vi "Wait for stop mMc Edited.vi"(5 "Controller #":string, 6 "wait for in pos":bool, 7 "Port":T1={"P type"=0, "reference"="", " Terminator "="\r\n", "Timeout"=300} {"Timeout" step=10; "P type" items=["none", "RS-232C"]}, 8 "error in (no error)":errorcluster) -> (0 "error out":errorcluster)   [LabVIEW 2021]
panel:
  out "Moving?":bool
  out "In position?":bool
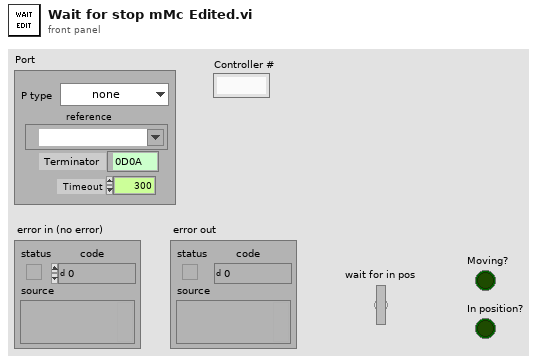
[diagram p1: front panel]
types:
  T1 = cluster{"P type":u16, "reference":refnum<visa-resource-name>, " Terminator ":string, "Timeout":i32}
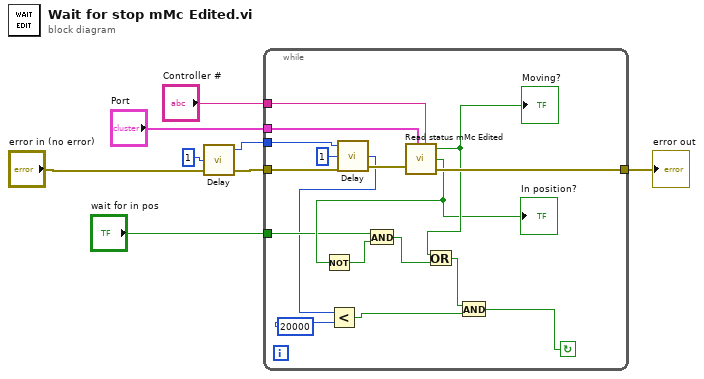
[diagram p0: block diagram]
diagram:
  n1 = call "Delay.vi"("milliseconds to wait"=u32 1, "error in (no error)"="error in (no error)") -> ("new time"=w1:u32, "error out"=w2:errorcluster)  [unwired: 5 in, 1 out]
  n2 = while {
    tunnel: "Port" -> [w25]
    tunnel: "Controller #" -> [w24]
    tunnel: [w23] -> w6
    tunnel: w2 -> [w16]
    tunnel: "wait for in pos" -> [w19]
    tunnel: w1 -> [w9]
    stop <- w10 continue-if-true
    n3 = call "Delay.vi"("old timer value"=w9, "milliseconds to wait"=u32 1, "error in (no error)"=w16) -> ("elapsed time"=w14:u32, "error out"=w15:errorcluster)  [unwired: 4 in, 1 out]
    n4 = Less?(x=w14, y=u32 20000) -> (x < y?=w11:bool)
    n5 = call "Read status mMc Edited.vi"("Port"=w25, "error in (no error)"=w15, "Controller #"=w24) -> ("Moving?"=w22:bool, "In position?"=w21:bool, "error out"=w23:errorcluster)  [unwired: 4 in]
    "Moving?" <- w22
    "In position?" <- w21
    n6 = Not(x=w21) -> (.not. x?=w18:bool)
    n7 = And(x=w19, y=w18) -> (x .and. y?=w20:bool)
    n8 = Or(x=w22, y=w20) -> (x .or. y?=w12:bool)
    n9 = And(x=w12, y=w11) -> (x .and. y?=w10:bool)
  }
  "error out" <- w6
